vi "Main.vi"() -> ()   [LabVIEW 2021]
doc: "Use this template to build a simple state machine design pattern. Each state executes code and determines which state to transition to."
uses:
  controls/State.ctl
  controls/Data.ctl
  vmmso/vmmso.lvlib
panel:
  out "Is IO Ready?":bool
  out "IO Read Return":u32 format="%x"
  out "IO4":bool
  out "IO0":bool
  in  "Amplitude":dbl=2000.0
  in  "Bias":dbl
  in  "Freq":dbl=1000.0
  in  "Wave Style":u16(ring) items=["Sine", "Square", "Ramp"]
  out "Is Data Ready？":bool
  out "ReadVoltageData Return":u32
  out "Voltage Wave":dbl[][](graph)
  out "Capture Return":i32
  out "Device is OK?":bool
  out "Support Samples":u32[](array[numeric])
  in  "Exit":bool
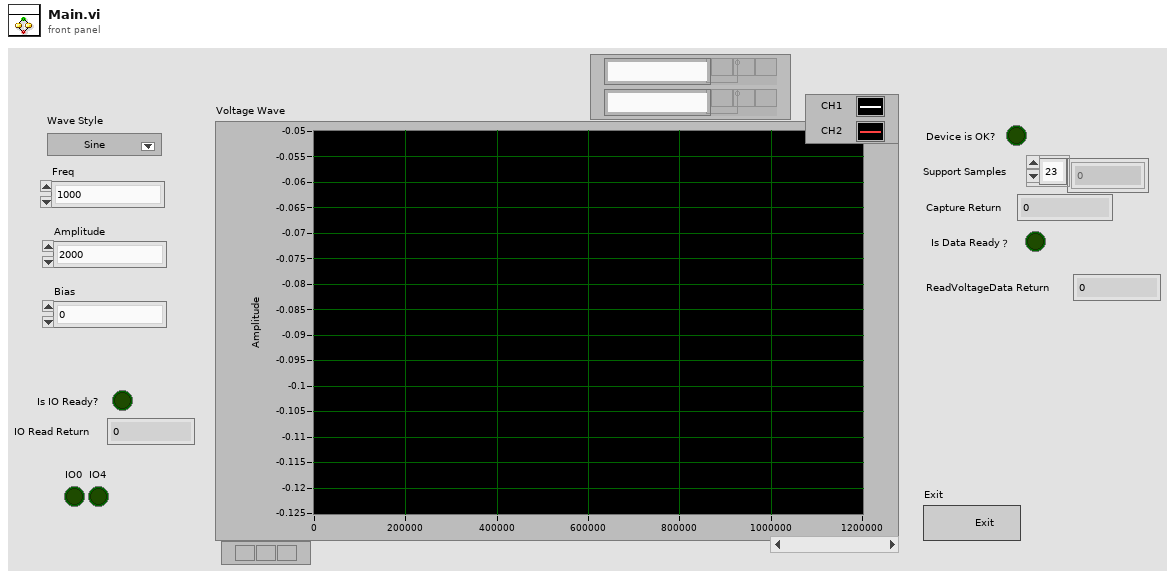
[diagram p1: front panel]
types:
  T1 = typedef "Data.ctl" = cluster{"Boolean <Exit Flag>":bool, "String <Replace Me>":string, "Numeric <Replace Me>":dbl}
  T2 = typedef "State.ctl" = enum16{"Initialize", "Wait for UsbIn", "Init Osc and Dds", "Wait for Event", "Capture", "Read Voltage", "Read IO", "Exit"}
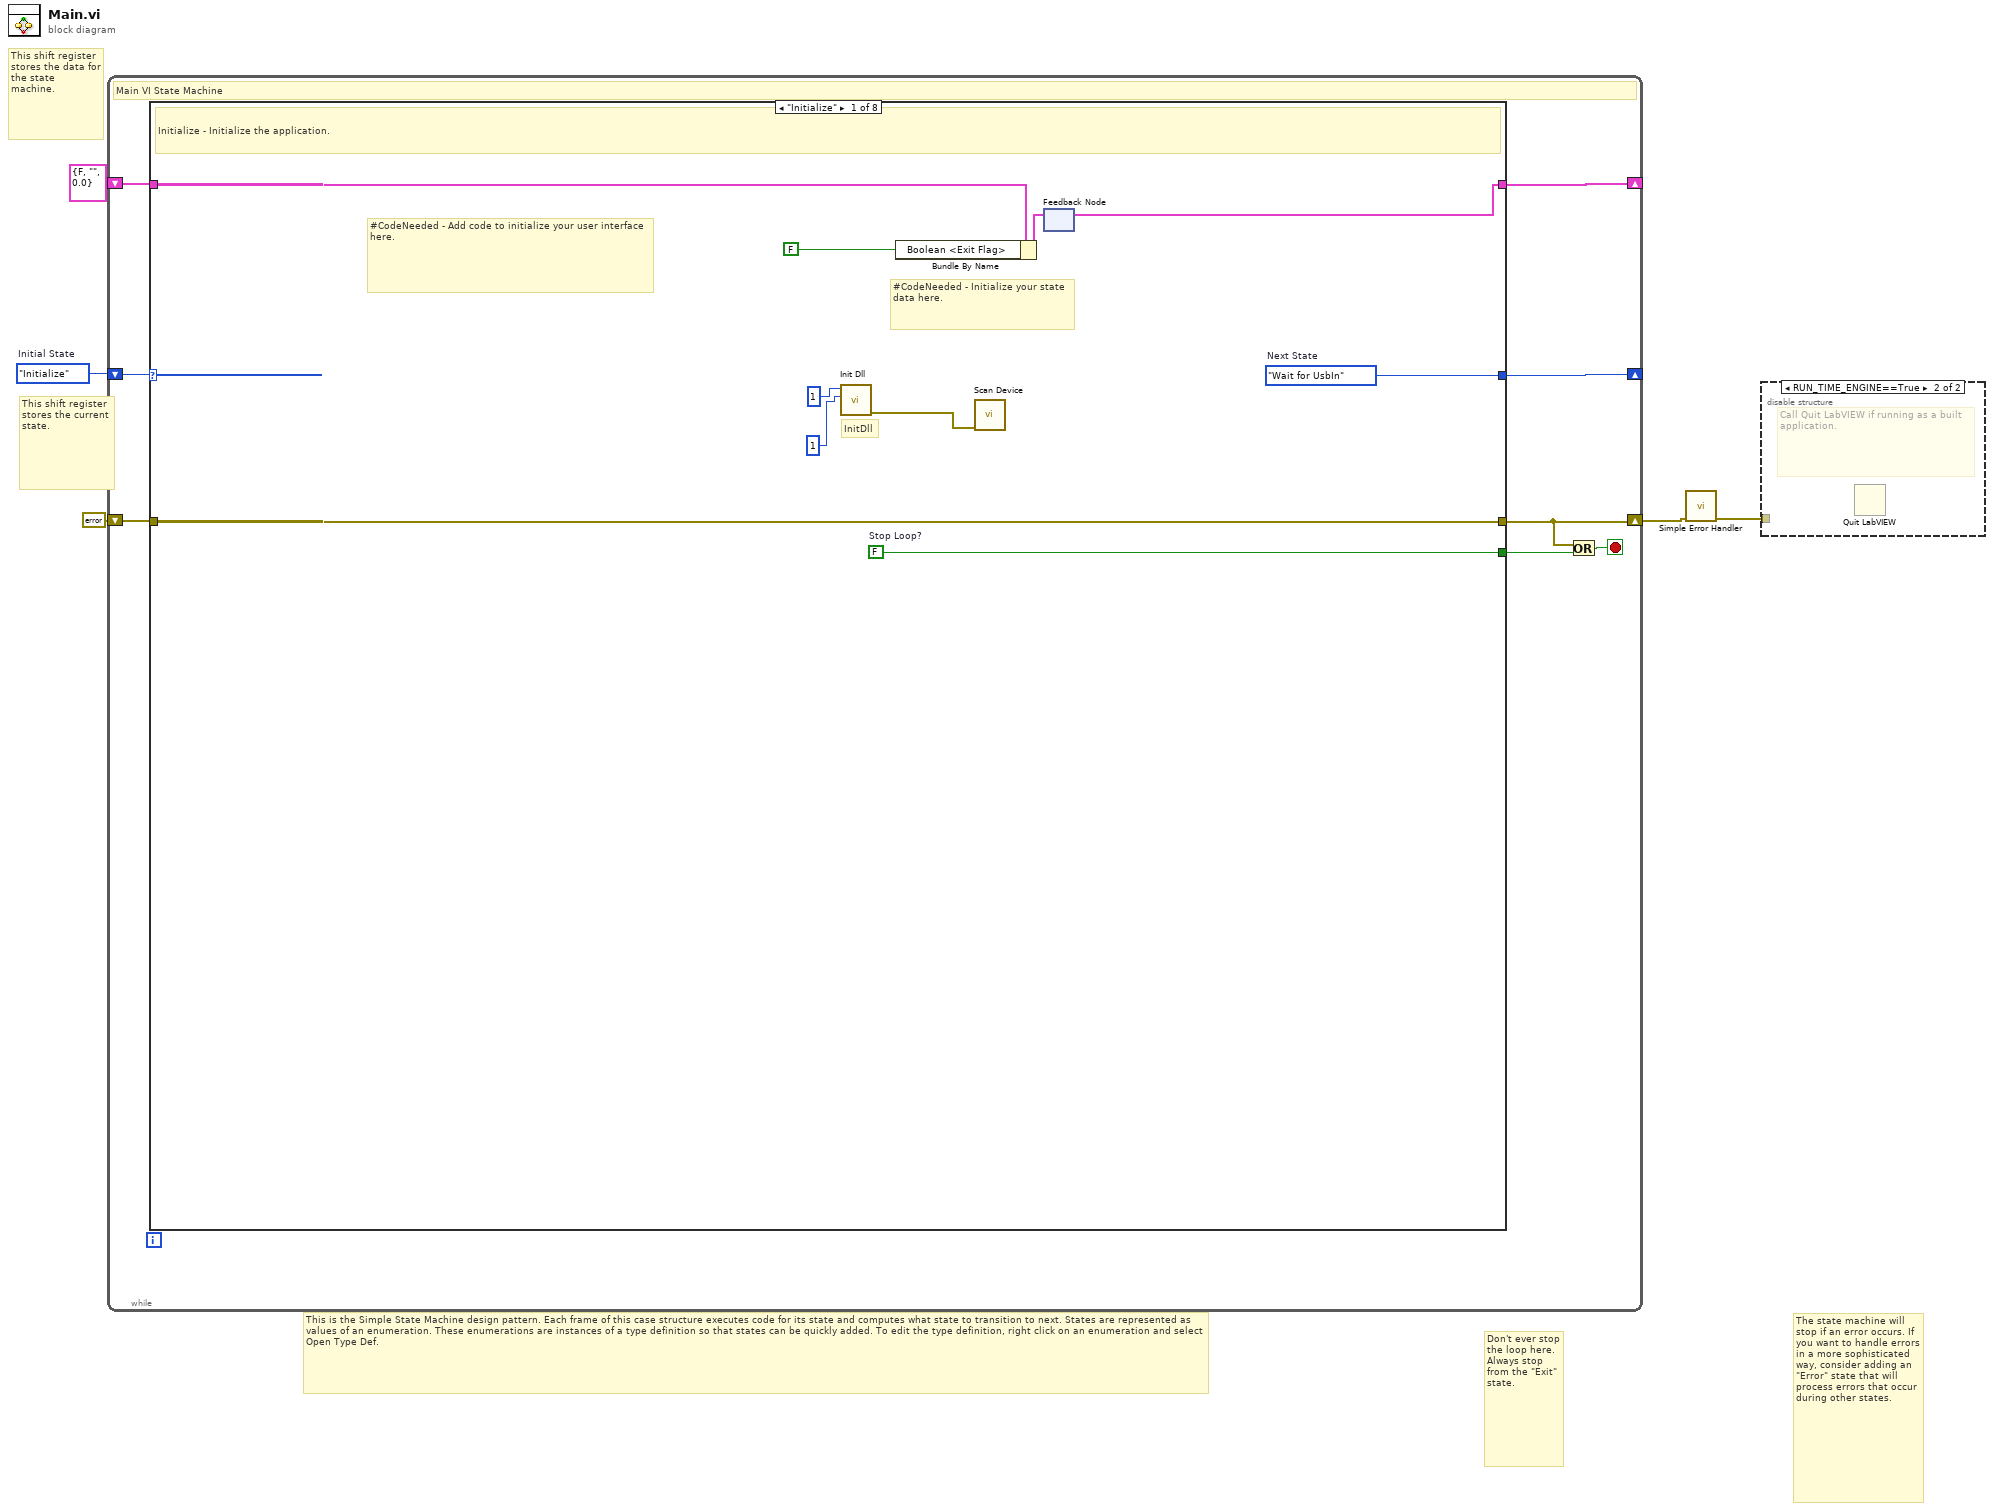
[diagram p0: block diagram]
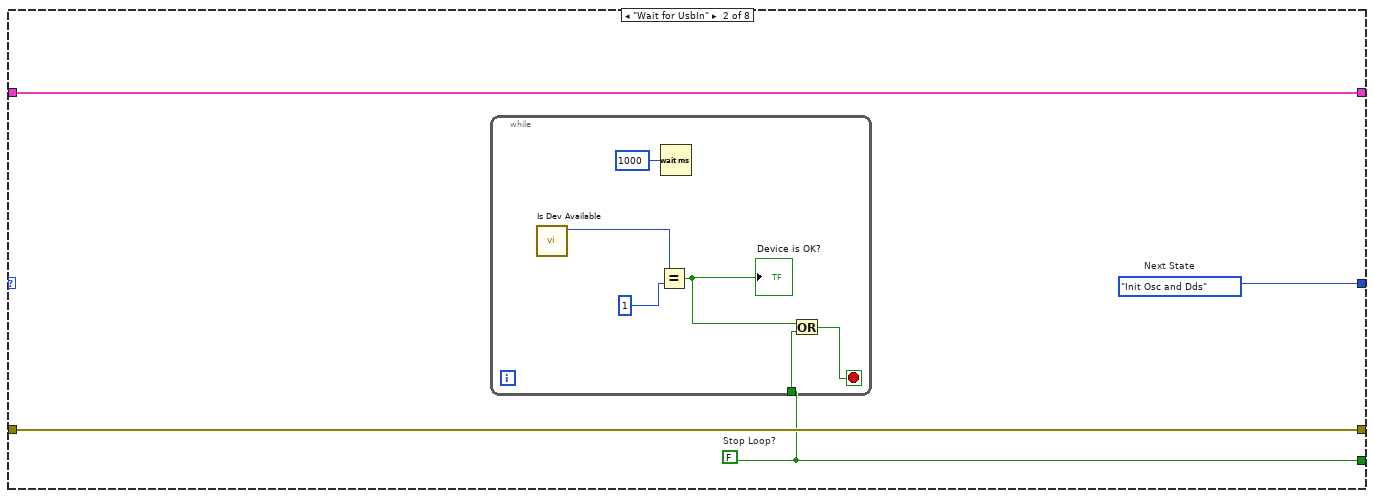
[diagram p3: hidden frame]
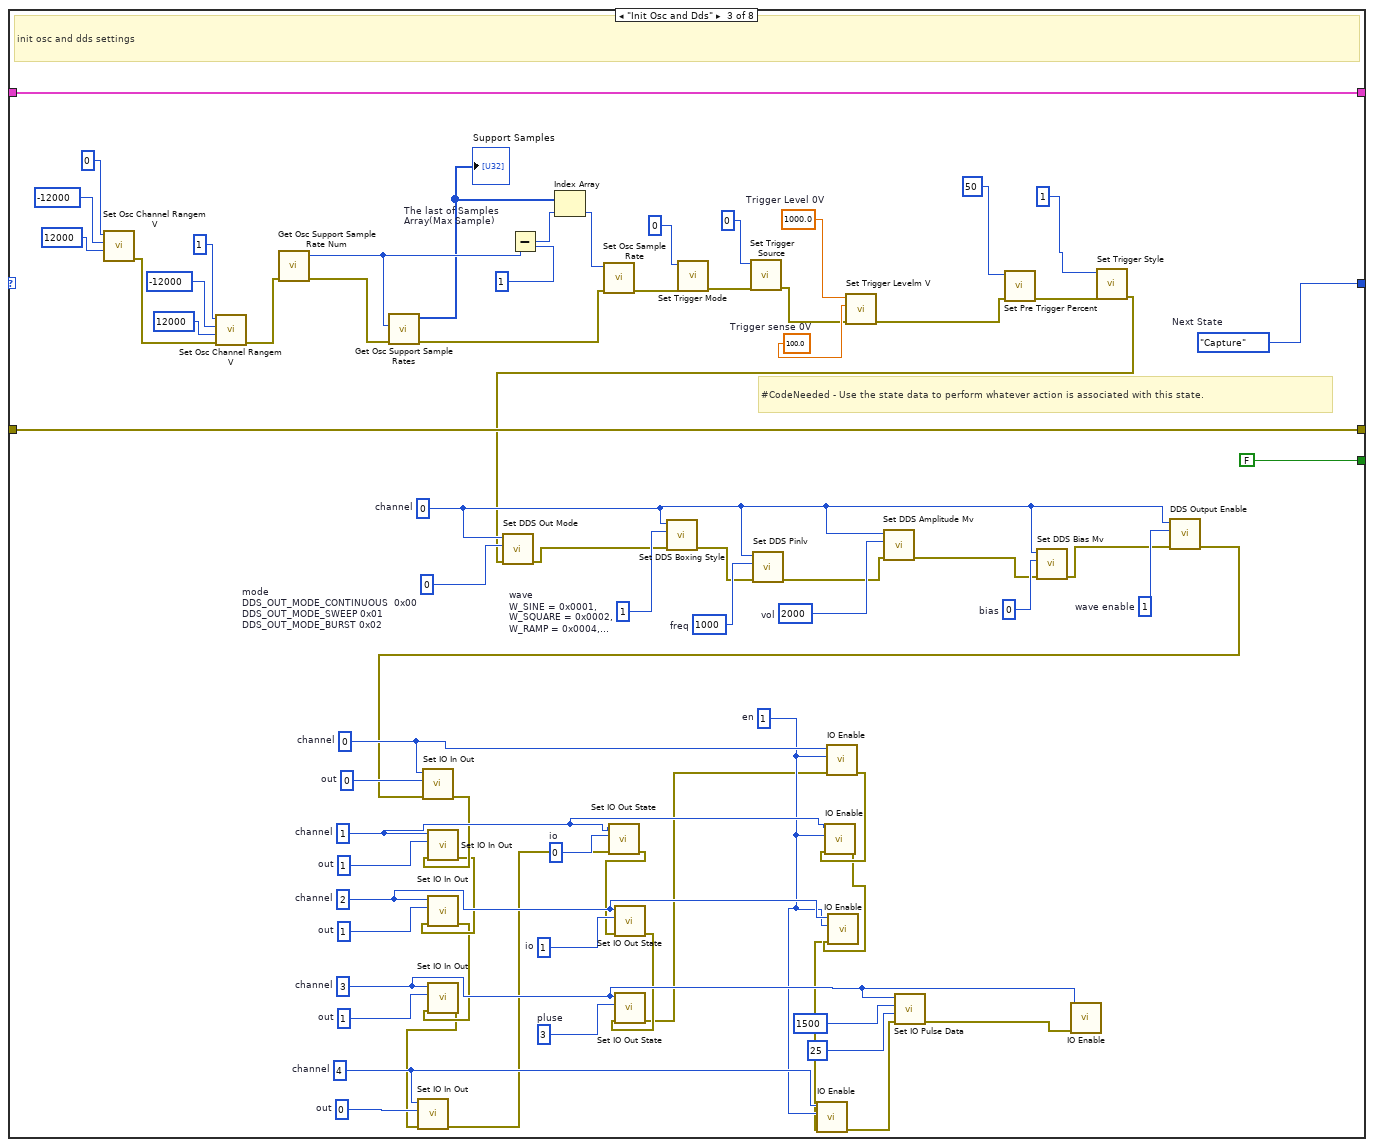
[diagram p4: hidden frame]
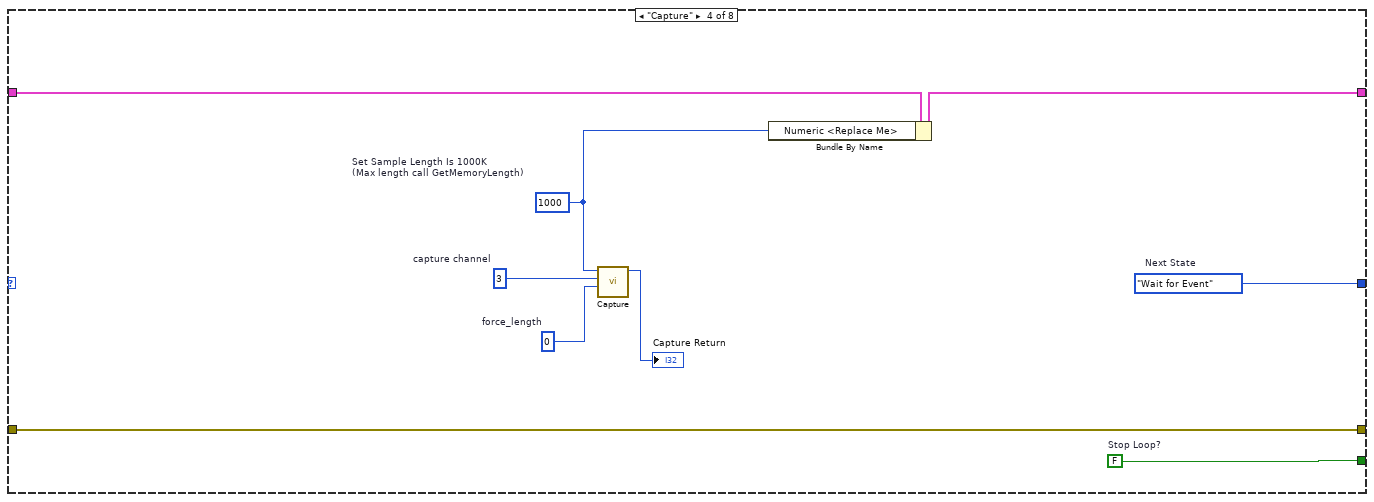
[diagram p5: hidden frame]
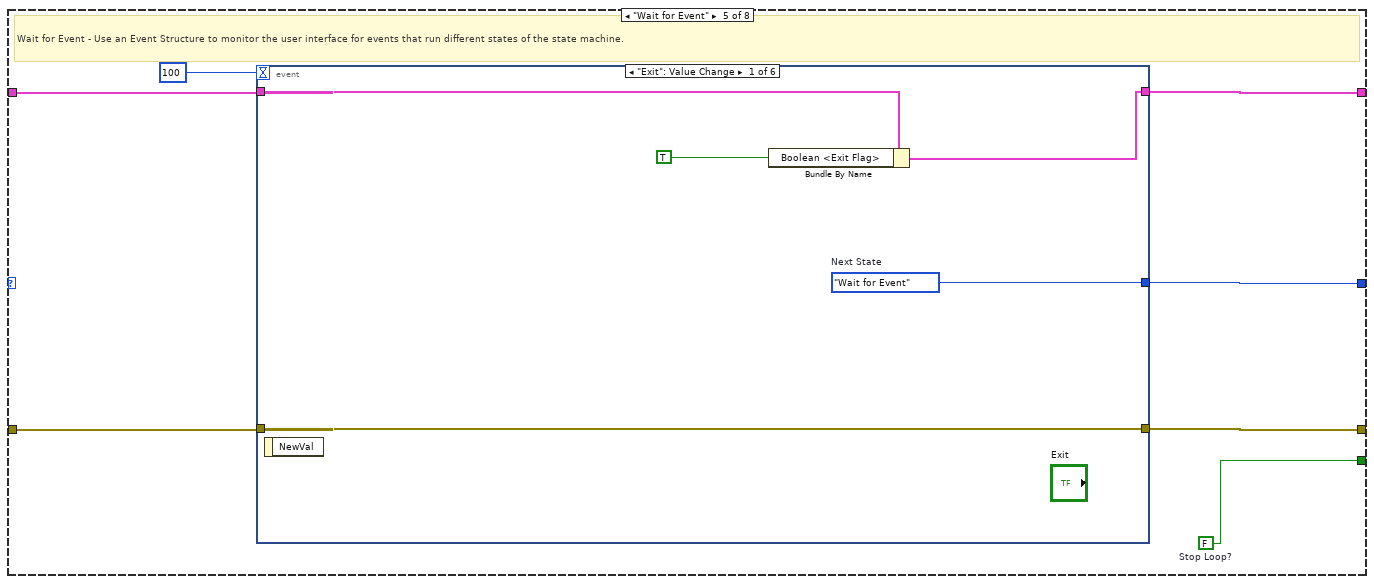
[diagram p6: hidden frame]
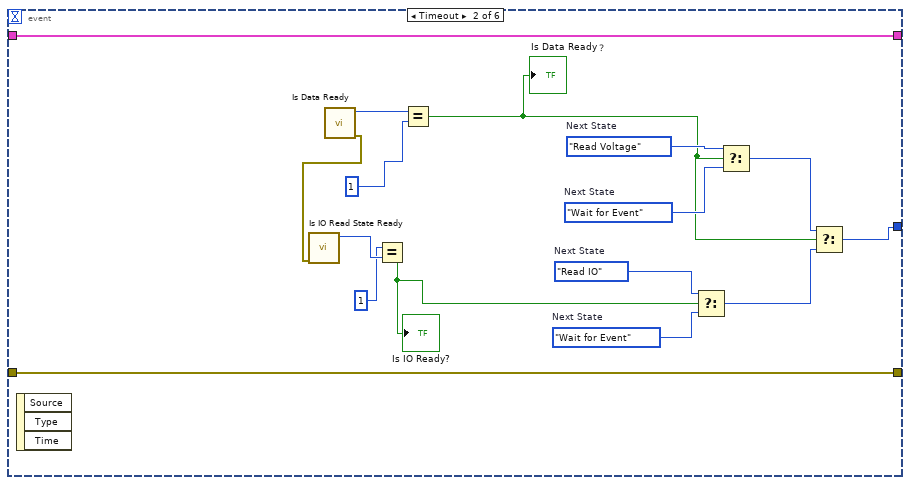
[diagram p7: hidden frame]
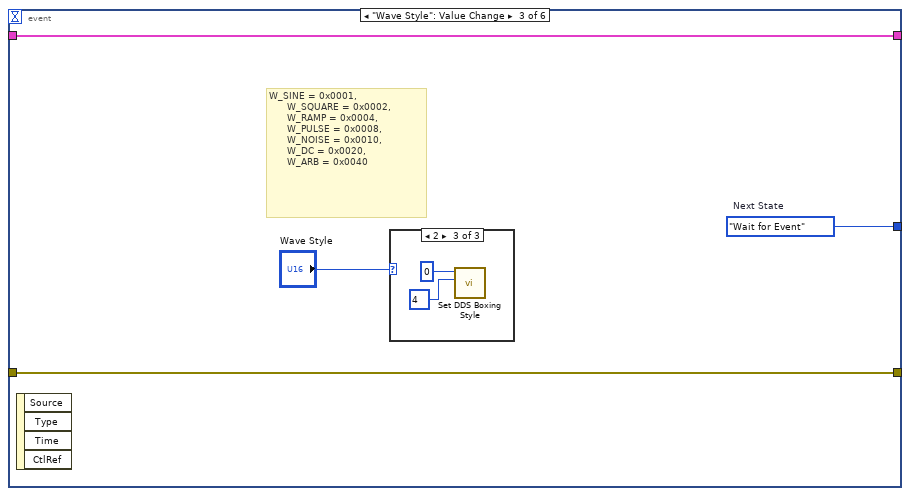
[diagram p8: hidden frame]
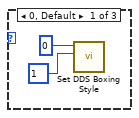
[diagram p9: hidden frame]
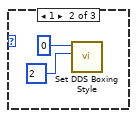
[diagram p10: hidden frame]
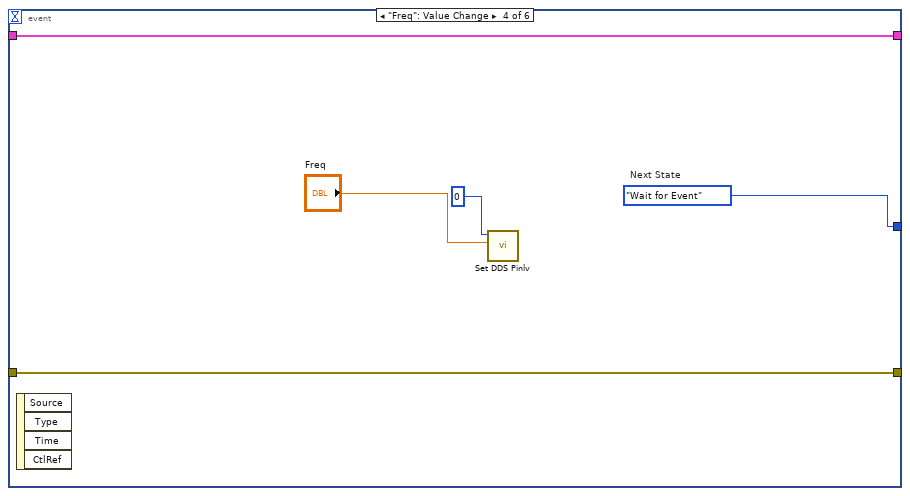
[diagram p11: hidden frame]
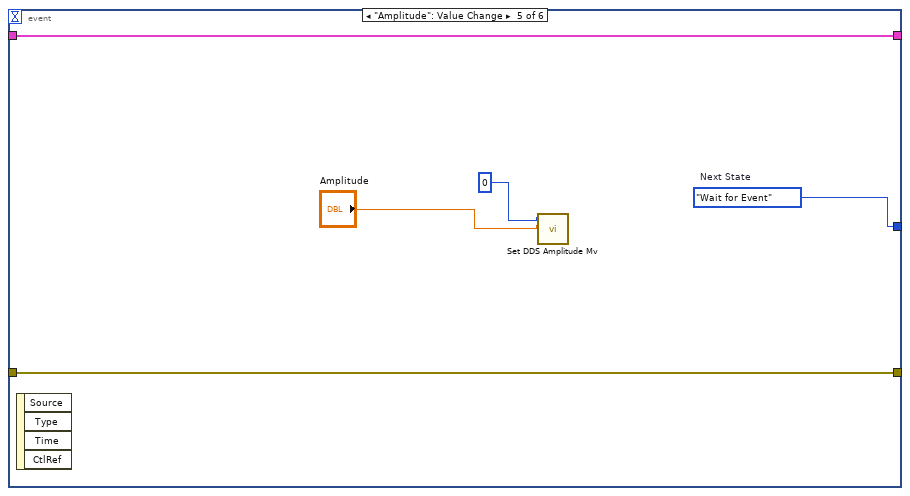
[diagram p12: hidden frame]
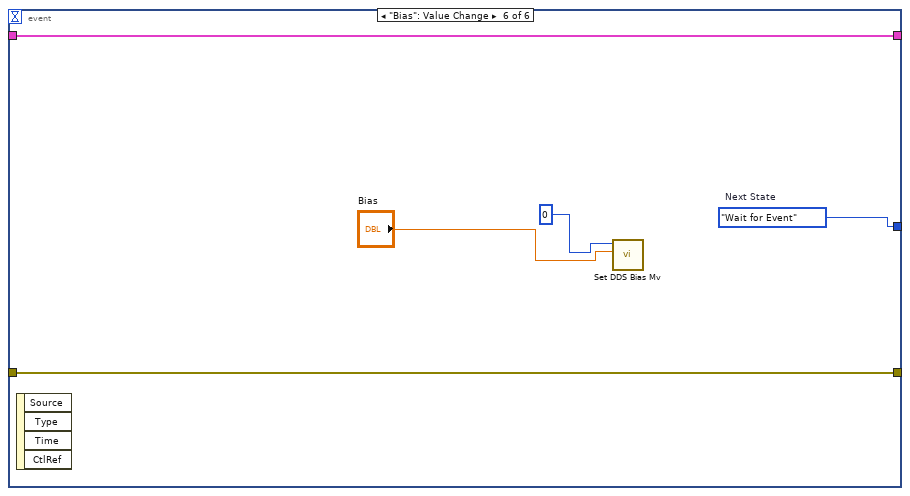
[diagram p13: hidden frame]
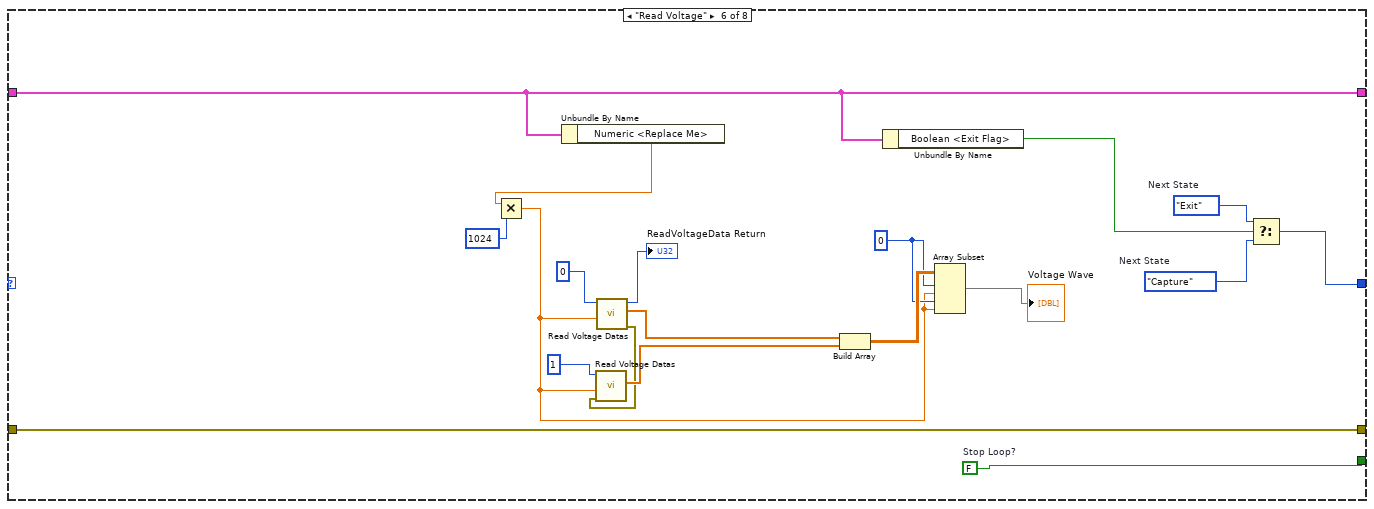
[diagram p14: hidden frame]
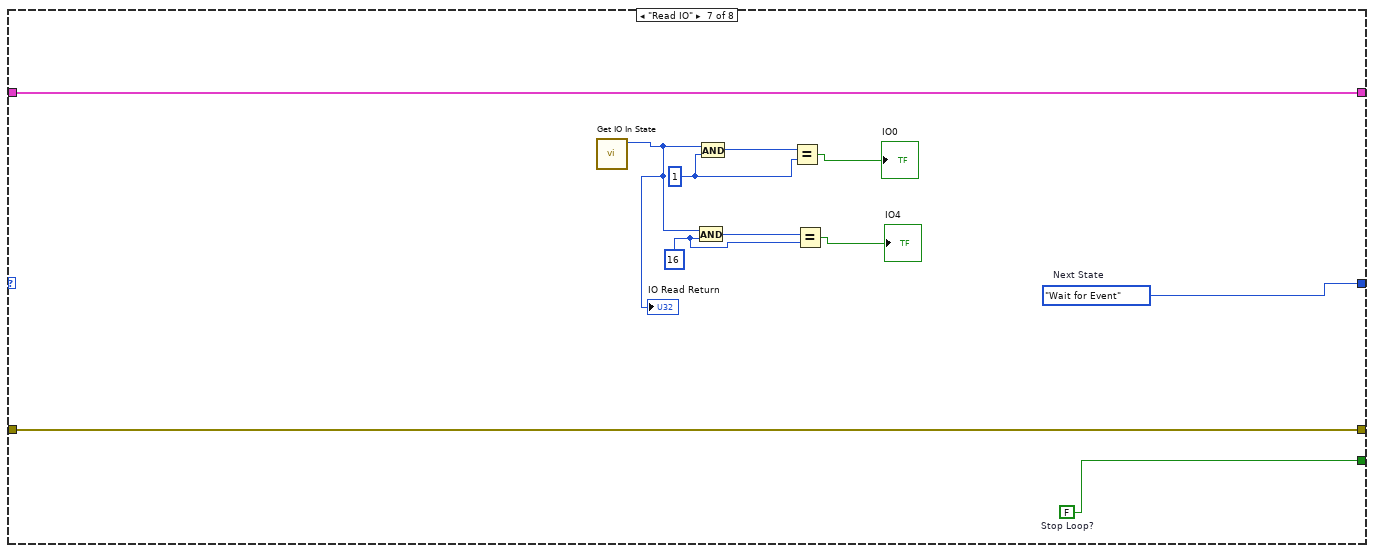
[diagram p15: hidden frame]
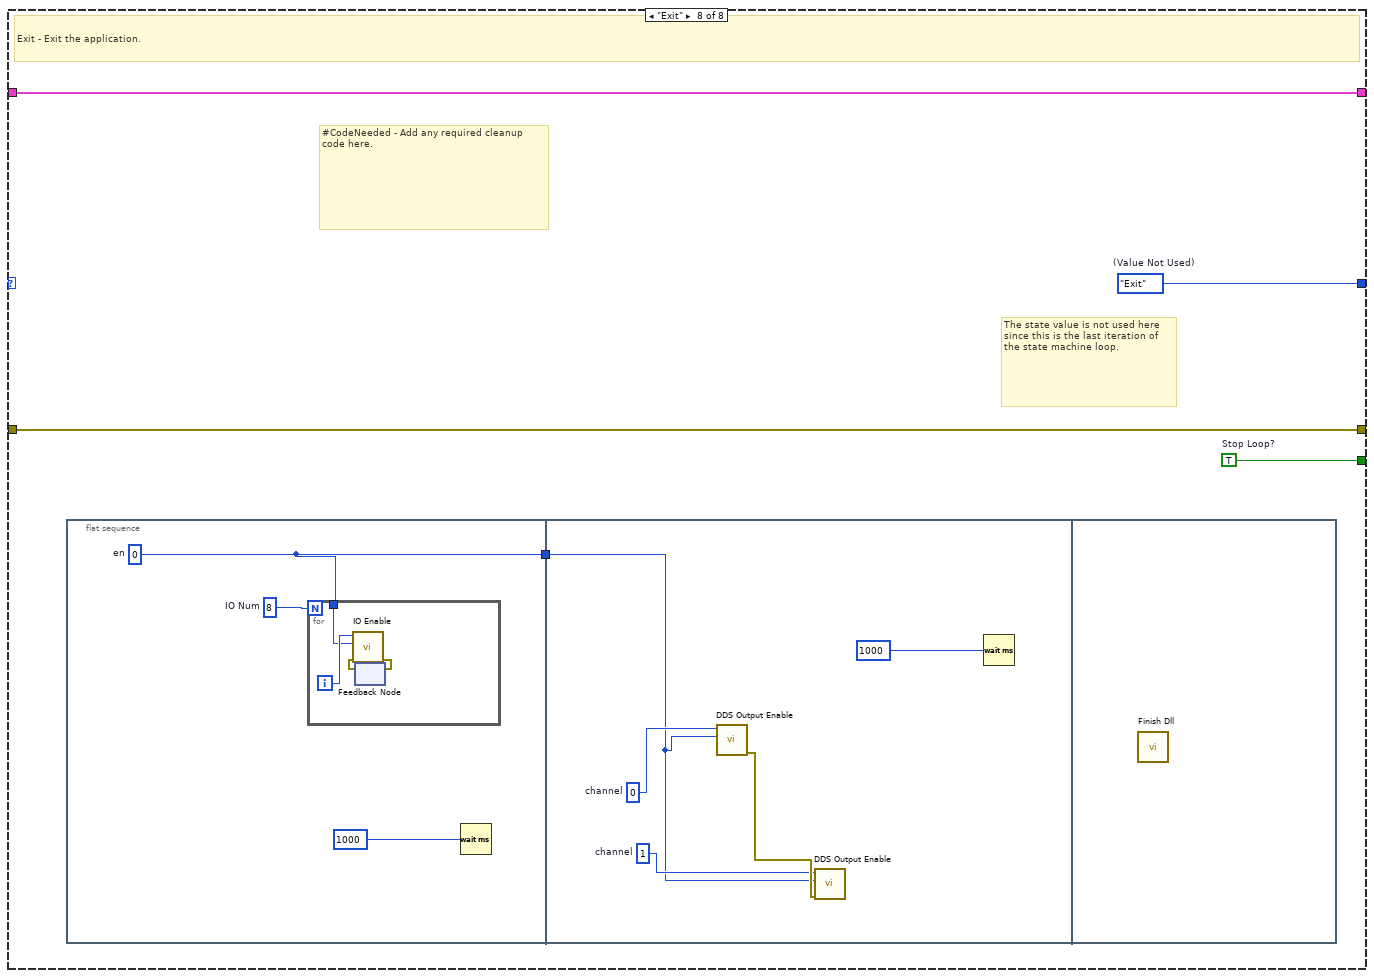
[diagram p16: hidden frame]
diagram:
  w5 = State."Initialize"  # Initial State
  # "Don't ever stop the loop here. Always stop from the \"Exit\" state."
  # "The state machine will stop if an error occurs. If you want to handle errors in a more sophisticated way, consider adding an \"Error\" state that will process errors that occur during other states."
  # "This shift register stores the data for the state machine."
  # "This is the Simple State Machine design pattern. Each frame of this case structure executes code for its state and computes what state to transition to next. States are represented as values of an enumeration. These enumerations are instances of a type definition so that states can be quickly added. To edit the type definition, right click on an enumeration and select Open Type Def."
  # "This shift register stores the current state."
  n1 = while {
    shift-right: [w12] -> _
    shift-left: w5 -> [w13]
    shift-right: [w10] -> _
    shift-left: T1 {"Boolean <Exit Flag>"=FALSE, "String <Replace Me>"="", "Numeric <Replace Me>"=0.0} ("Data") -> [w11]
    shift-right: [w7] -> w2
    shift-left: errorcluster {"status"=FALSE, "code"=0, "source"=""} ("error constant") -> [w9]
    stop <- w8 stop-if-true
    # "Main VI State Machine"
    n2 = case shown="\"Initialize\"" w13 {
      tunnel: [w23 w26 w106 w114 w122 w170 w189 w203] -> w12
      tunnel: w11 -> [w14 w24 w104 w109 w121 w174 w198 w202]
      tunnel: [w15 w24 w104 w108 w120 w174 w198 w202] -> w10
      tunnel: w9 -> [w21 w27 w103 w115 w119 w187 w197 w200]
      tunnel: [w21 w27 w103 w115 w118 w187 w197 w200] -> w7
      tunnel: [w22 w25 FALSE ("Stop Loop?") w113 w116 w186 w188 w201] -> w6
      frame "Initialize" {
        w22 = FALSE  # Stop Loop?
        w23 = State."Wait for UsbIn"  # Next State
        # "InitDll"
        # "#CodeNeeded - Initialize your state data here."
        # "#CodeNeeded - Add code to initialize your user interface here."
        # "Initialize - Initialize the application."
        n3 = call "Init Dll.vi"("en_hard_watchdog"=1 ("channel"), "en_log"=1 ("channel")) -> ("error out"=w18:errorcluster)  [unwired: 8 in, 1 out]
        n4 = Bundle By Name(cluster=w14, "Boolean <Exit Flag>"=FALSE) -> (w16:T1)
        n5 = call "Scan Device.vi"("error in (no error)"=w18) -> ()  [unwired: 9 in, 2 out]
        n6 = feedback-in #1(w16) -> ()
        n7 = feedback #1() -> (w15:T1)  [unwired: 1 in]
      }
      frame "Wait for UsbIn" {
        w26 = State."Init Osc and Dds"  # Next State
        w25 = FALSE  # Stop Loop?
        n8 = while {
          tunnel: w25 -> [w31]
          stop <- w30 stop-if-true
          n9 = call "Is Dev Available.vi"() -> ("function return"=w29:i32)  [unwired: 10 in, 1 out]
          n10 = Equal?(x=w29, y=1 ("channel")) -> (x = y?=w28:bool)
          "Device is OK?" <- w28
          n11 = Wait (ms)(milliseconds to wait=u32 1000 ("等待时间（毫秒）")) -> ()  [unwired: 1 out]
          n12 = Or(x=w28, y=w31) -> (x .or. y?=w30:bool)
        }
      }
      frame "Init Osc and Dds" {
        w65 = i8 0  # out
        w64 = i8 4  # channel
        w69 = i8 3  # pluse
        w70 = i8 1  # out
        w68 = i8 3  # channel
        w63 = i8 1  # en
        w74 = i8 0  # io
        w75 = i8 1  # io
        w76 = i8 1  # out
        w71 = i8 2  # channel
        w77 = i8 1  # out
        w72 = i8 1  # channel
        w78 = i8 0  # out
        w73 = i8 0  # channel
        w79 = sgl 100.0  # Trigger sense 0V
        w84 = i8 0  # mode DDS_OUT_MODE_CONTINUOUS  0x00 DDS_OUT_MODE_SWEEP 0x01 DDS_OUT_MODE_BURST 0x02
        w86 = i8 1  # wave enable
        w88 = u32 0  # bias
        w87 = u32 2000  # vol
        w89 = u32 1000  # freq
        w90 = i8 1  # wave  W_SINE = 0x0001,  W_SQUARE = 0x0002,  W_RAMP = 0x0004,  W_PULSE = 0x0008,  W_NOISE = 0x0010,  W_DC = 0x0020,  W_ARB = 0x0040
        w85 = i8 0  # channel
        w80 = sgl 1000.0  # Trigger Level 0V
        w106 = State."Capture"  # Next State
        # "#CodeNeeded - Use the state data to perform whatever action is associated with this state."
        # "init osc and dds settings"
        n13 = call "Set Osc Channel Rangem V.vi"("maxmv"=12000 ("minmv"), "minmv"=-12000, "channel"=0) -> ("error out"=w62:errorcluster)  [unwired: 7 in, 1 out]
        n14 = call "Set Osc Channel Rangem V.vi"("error in (no error)"=w62, "maxmv"=12000 ("minmv"), "minmv"=-12000, "channel"=1) -> ("error out"=w61:errorcluster)  [unwired: 6 in, 1 out]
        n15 = call "Get Osc Support Sample Rate Num.vi"("error in (no error)"=w61) -> ("error out"=w60:errorcluster, "function return"=w95:i32)  [unwired: 9 in]
        n16 = call "Get Osc Support Sample Rates.vi"("error in (no error)"=w60, "maxnum"=w95) -> ("error out"=w59:errorcluster, "sample out"=w92:u32[])  [unwired: 7 in, 1 out]
        "Support Samples" <- w92
        n17 = Subtract "The last of Samples Array(Max Sample)"(x=w95, y=1 ("front")) -> (x-y=w97:i32)
        n18 = Index Array(array=w92, index=w97) -> (element=w98:u32)
        n19 = call "Set Osc Sample Rate.vi"("error in (no error)"=w59, "sample"=w98) -> ("error out"=w58:errorcluster)  [unwired: 8 in, 1 out]
        n20 = call "Set Trigger Mode.vi"("error in (no error)"=w58, "mode"=0 ("front")) -> ("error out"=w57:errorcluster)  [unwired: 9 in]
        n21 = call "Set Trigger Source.vi"("error in (no error)"=w57, "source"=0 ("front")) -> ("error out"=w56:errorcluster)  [unwired: 9 in]
        n22 = call "Set Trigger Levelm V.vi"("error in (no error)"=w56, "sense_mv"=w79, "level_mv"=w80) -> ("error out"=w55:errorcluster)  [unwired: 8 in]
        n23 = call "Set Pre Trigger Percent.vi"("error in (no error)"=w55, "front"=50) -> ("error out"=w54:errorcluster)  [unwired: 9 in]
        n24 = call "Set Trigger Style.vi"("error in (no error)"=w54, "style"=u32 1) -> ("error out"=w34:errorcluster)  [unwired: 9 in]
        n25 = call "Set DDS Out Mode.vi"("error in (no error)"=w34, "out_mode"=w84, "channel_index"=w85) -> ("error out"=w53:errorcluster)  [unwired: 8 in]
        n26 = call "Set DDS Boxing Style.vi"("error in (no error)"=w53, "boxing"=w90, "channel_index"=w85) -> ("error out"=w52:errorcluster)  [unwired: 8 in]
        n27 = call "Set DDS Pinlv.vi"("error in (no error)"=w52, "pinlv"=w89, "channel_index"=w85) -> ("error out"=w51:errorcluster)  [unwired: 8 in]
        n28 = call "Set DDS Amplitude Mv.vi"("error in (no error)"=w51, "amplitdude"=w87, "channel_index"=w85) -> ("error out"=w50:errorcluster)  [unwired: 8 in]
        n29 = call "Set DDS Bias Mv.vi"("error in (no error)"=w50, "bias"=w88, "channel_index"=w85) -> ("error out"=w49:errorcluster)  [unwired: 8 in]
        n30 = call "DDS Output Enable.vi"("error in (no error)"=w49, "enable"=w86, "channel_index"=w85) -> ("error out"=w35:errorcluster)  [unwired: 8 in]
        n31 = call "Set IO In Out.vi"("error in (no error)"=w35, "inout"=w78, "channel"=w73) -> ("error out"=w48:errorcluster)  [unwired: 8 in]
        n32 = call "Set IO In Out.vi"("error in (no error)"=w48, "inout"=w77, "channel"=w72) -> ("error out"=w47:errorcluster)  [unwired: 8 in]
        n33 = call "Set IO In Out.vi"("error in (no error)"=w47, "inout"=w76, "channel"=w71) -> ("error out"=w46:errorcluster)  [unwired: 8 in]
        n34 = call "Set IO In Out.vi"("error in (no error)"=w46, "inout"=w70, "channel"=w68) -> ("error out"=w45:errorcluster)  [unwired: 8 in]
        n35 = call "Set IO In Out.vi"("error in (no error)"=w45, "inout"=w65, "channel"=w64) -> ("error out"=w44:errorcluster)  [unwired: 8 in]
        n36 = call "Set IO Out State.vi"("error in (no error)"=w44, "state"=w74, "channel"=w72) -> ("error out"=w43:errorcluster)  [unwired: 8 in]
        n37 = call "Set IO Out State.vi"("error in (no error)"=w43, "state"=w75, "channel"=w71) -> ("error out"=w42:errorcluster)  [unwired: 8 in]
        n38 = call "Set IO Out State.vi"("error in (no error)"=w42, "state"=w69, "channel"=w68) -> ("error out"=w41:errorcluster)  [unwired: 8 in]
        n39 = call "IO Enable.vi"("error in (no error)"=w41, "enable"=w63, "channel"=w73) -> ("error out"=w40:errorcluster)  [unwired: 8 in]
        n40 = call "IO Enable.vi"("error in (no error)"=w40, "enable"=w63, "channel"=w72) -> ("error out"=w39:errorcluster)  [unwired: 8 in]
        n41 = call "IO Enable.vi"("error in (no error)"=w39, "enable"=w63, "channel"=w71) -> ("error out"=w38:errorcluster)  [unwired: 8 in]
        n42 = call "IO Enable.vi"("error in (no error)"=w38, "enable"=w63, "channel"=w64) -> ("error out"=w37:errorcluster)  [unwired: 8 in]
        n43 = call "Set IO Pulse Data.vi"("error in (no error)"=w37, "duty"=25 ("minmv"), "hz"=1500 ("minmv"), "channel"=w68) -> ("error out"=w36:errorcluster)  [unwired: 7 in]
        n44 = call "IO Enable.vi"("error in (no error)"=w36, "channel"=w68) -> ()  [unwired: 9 in, 1 out]
      }
      frame "Capture" {
        w110 = i8 0  # force_length
        w107 = u32 1000  # Set Sample Length Is 1000K (Max length call GetMemoryLength)
        w111 = i8 3  # capture channel
        w113 = FALSE  # Stop Loop?
        w114 = State."Wait for Event"  # Next State
        n45 = call "Capture.vi"("force_length"=w110, "capture_channel"=w111, "length"=w107) -> ("function return"=→"Capture Return":i32)  [unwired: 7 in, 1 out]
        n46 = Bundle By Name(cluster=w109, "Numeric <Replace Me>"=w107) -> (w108:T1)
      }
      frame "Wait for Event" {
        w116 = FALSE  # Stop Loop?
        # "Wait for Event - Use an Event Structure to monitor the user interface for events that run different states of the state machine."
        n47 = event shown="[0] \"Exit\": Value Change" {
          selector: _ -> [_ _ _ _ _ _]
          dyn-events: _ -> [_ _ _ _ _ _]
          timeout: 100 ("y") -> [_ _ _ _ _ _]
          tunnel: [w127 w132 w144 w156 w161 w166] -> w122
          tunnel: w121 -> [w125 w143 w147 w158 w163 w168]
          tunnel: [w124 w143 w147 w158 w163 w168] -> w120
          tunnel: w119 -> [w126 w142 w146 w157 w162 w167]
          tunnel: [w126 w142 w146 w157 w162 w167] -> w118
          event "Exit": Value Change {
            w127 = State."Wait for Event"  # Next State
            n48 = event-data() -> ()  [unwired: 1 in, 1 out]
            n49 = Bundle By Name(cluster=w125, "Boolean <Exit Flag>"=TRUE) -> (w124:T1)
          }
          event Timeout {
            w134 = State."Wait for Event"  # Next State
            w135 = State."Read IO"  # Next State
            w139 = State."Wait for Event"  # Next State
            w140 = State."Read Voltage"  # Next State
            n50 = event-data() -> ()  [unwired: 1 in, 3 out]
            n51 = call "Is Data Ready.vi"() -> ("error out"=w128:errorcluster, "function return"=w141:i32)  [unwired: 10 in]
            n52 = call "Is IO Read State Ready.vi"("error in (no error)"=w128) -> ("function return"=w137:i32)  [unwired: 9 in, 1 out]
            n53 = Equal?(x=1 ("y"), y=w137) -> (x = y?=w136:bool)
            "Is IO Ready?" <- w136
            n54 = Equal?(x=w141, y=1) -> (x = y?=w131:bool)
            "Is Data Ready？" <- w131
            n55 = Select(t=w135, s=w136, f=w134) -> (s? t:f=w129:T2)
            n56 = Select(t=w140, s=w131, f=w139) -> (s? t:f=w130:T2)
            n57 = Select(t=w130, s=w131, f=w129) -> (s? t:f=w132:T2)
          }
          event "Wave Style": Value Change {
            w144 = State."Wait for Event"  # Next State
            # "W_SINE = 0x0001, \n\t\t\t\t\t\tW_SQUARE = 0x0002, \n\t\t\t\t\t\tW_RAMP = 0x0004, \n\t\t\t\t\t\tW_PULSE = 0x0008, \n\t\t\t\t\t\tW_NOISE = 0x0010, \n\t\t\t\t\t\tW_DC = 0x0020, \n\t\t\t\t\t\tW_ARB = 0x0040"
            n58 = event-data() -> ()  [unwired: 1 in, 4 out]
            n59 = case shown="2" "Wave Style" {
              frame 0, Default {
                n60 = call "Set DDS Boxing Style.vi"("boxing"=1 ("y"), "channel_index"=0 ("y")) -> ()  [unwired: 9 in, 1 out]
              }
              frame 1 {
                n61 = call "Set DDS Boxing Style.vi"("boxing"=2 ("y"), "channel_index"=0 ("y")) -> ()  [unwired: 9 in, 1 out]
              }
              frame 2 {
                n62 = call "Set DDS Boxing Style.vi"("boxing"=4 ("y"), "channel_index"=0 ("y")) -> ()  [unwired: 9 in, 1 out]
              }
            }
          }
          event "Freq": Value Change {
            w156 = State."Wait for Event"  # Next State
            n63 = event-data() -> ()  [unwired: 1 in, 4 out]
            n64 = call "Set DDS Pinlv.vi"("pinlv"="Freq", "channel_index"=0 ("y")) -> ()  [unwired: 9 in, 1 out]
          }
          event "Amplitude": Value Change {
            w161 = State."Wait for Event"  # Next State
            n65 = event-data() -> ()  [unwired: 1 in, 4 out]
            n66 = call "Set DDS Amplitude Mv.vi"("amplitdude"="Amplitude", "channel_index"=0 ("y")) -> ()  [unwired: 9 in, 1 out]
          }
          event "Bias": Value Change {
            w166 = State."Wait for Event"  # Next State
            n67 = event-data() -> ()  [unwired: 1 in, 4 out]
            n68 = call "Set DDS Bias Mv.vi"("bias"="Bias", "channel_index"=0 ("y")) -> ()  [unwired: 9 in, 1 out]
          }
        }
      }
      frame "Read Voltage" {
        w172 = State."Exit"  # Next State
        w176 = i8 0 ("channel")
        w171 = State."Capture"  # Next State
        w186 = FALSE  # Stop Loop?
        n69 = Unbundle By Name(w174) -> ("Numeric <Replace Me>"=w182:dbl)
        n70 = Multiply(x=w182, y=1024) -> (x*y=w175:dbl)
        n71 = call "Read Voltage Datas.vi"("length"=w175, "channel"=i8 0) -> ("error out"=w169:errorcluster, "buffer out"=w180:dbl[], "function return"=→"ReadVoltageData Return":u32)  [unwired: 7 in]
        n72 = call "Read Voltage Datas.vi"("error in (no error)"=w169, "length"=w175, "channel"=i8 1) -> ("buffer out"=w179:dbl[])  [unwired: 6 in, 2 out]
        n73 = Build Array(w180, w179) -> (w178:dbl[][])
        n74 = Unbundle By Name(w174) -> ("Boolean <Exit Flag>"=w173:bool)
        n75 = Array Subset(array=w178, index (row)=w176, length (row)=w175, index (col)=w176, length (col)=w175) -> (→"Voltage Wave":dbl[][])
        n76 = Select(t=w172, s=w173, f=w171) -> (s? t:f=w170:T2)
      }
      frame "Read IO" {
        w188 = FALSE  # Stop Loop?
        w189 = State."Wait for Event"  # Next State
        w195 = 16 ("front")
        w192 = 1 ("front")
        n77 = call "Get IO In State.vi"() -> ("function return"=w191:u32)  [unwired: 10 in, 1 out]
        "IO Read Return" <- w191
        n78 = And(x=w191, y=w195) -> (x .and. y?=w194:u32)
        n79 = And(x=w191, y=w192) -> (x .and. y?=w190:u32)
        n80 = Equal?(x=w190, y=w192) -> (x = y?=→"IO0":bool)
        n81 = Equal?(x=w194, y=w195) -> (x = y?=→"IO4":bool)
      }
      frame "Exit" {
        w201 = TRUE  # Stop Loop?
        w203 = State."Exit"  # (Value Not Used)
        # "#CodeNeeded - Add any required cleanup code here."
        # "The state value is not used here since this is the last iteration of the state machine loop."
        # "Exit - Exit the application."
        n82 = flat-sequence {
          tunnel: [w205] -> w199
          tunnel: w199 -> [w212]
          frame #0 {
            w206 = i8 8  # IO Num
            w205 = i8 0  # en
            n83 = for {
              N: w206 -> [_]
              tunnel: w205 -> [w209]
              i -> [w210]
              n84 = feedback #2() -> (w207:errorcluster)  [unwired: 1 in]
              n85 = call "IO Enable.vi"("error in (no error)"=w207, "enable"=w209, "channel"=w210) -> ("error out"=w208:errorcluster)  [unwired: 8 in]
              n86 = feedback-in #2(w208) -> ()
            }
            n87 = Wait (ms)(milliseconds to wait=1000) -> ()  [unwired: 1 out]
          }
          frame #1 {
            w214 = i8 1  # channel
            w213 = i8 0  # channel
            n88 = call "DDS Output Enable.vi"("enable"=w212, "channel_index"=w213) -> ("error out"=w215:errorcluster)  [unwired: 9 in]
            n89 = call "DDS Output Enable.vi"("error in (no error)"=w215, "enable"=w212, "channel_index"=w214) -> ()  [unwired: 8 in, 1 out]
            n90 = Wait (ms)(milliseconds to wait=1000) -> ()  [unwired: 1 out]
          }
          frame #2 {
            n91 = call "Finish Dll.vi"() -> ()  [unwired: 10 in, 2 out]
          }
        }
      }
    }
    n92 = Or(x=w7, y=w6) -> (x .or. y?=w8:bool)
  }
  n93 = call <vilib>:"Simple Error Handler.vi"("error in (no error)"=w2) -> ("error out"=w1:errorcluster)  [unwired: 4 in, 4 out]
  n94 = disable-structure shown="RUN_TIME_ENGINE==True" {
    disable-tunnel: w1 -> [_ _]
    frame condition #0 (active) {
    }
    frame condition #1 {
      # "Call Quit LabVIEW if running as a built application."
      n95 = Quit LabVIEW() -> ()  [unwired: 1 in]
    }
  }
